vi "SnapShoot.vi"(8 "error in (no error)":errorcluster, 11 "ICameraTestingProxy in":refnum<class "ICameraTestingProxy.lvclass">) -> (0 "error out":errorcluster, 2 "SnapData":T1, 3 "ICameraTestingProxy out":refnum<class "ICameraTestingProxy.lvclass">)   [LabVIEW 2020, in "ICameraTestingProxy.lvlib" / "ICameraTestingProxy.lvclass"]
uses:
  ICameraTestingProxy.lvclass
  TypeDef/SnapData.ctl
  TypeDef/ICameraTestingProxy_typedef.lvlib
  TypeDef/Resolution.ctl
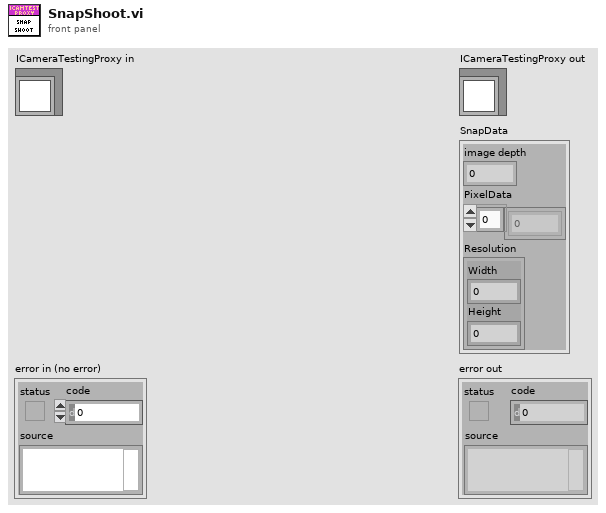
[diagram p1: front panel]
types:
  T1 = typedef "ICameraTestingProxy_typedef.lvlib/SnapData.ctl" = cluster{"image depth":i32, "PixelData":u8[], "Resolution":T2}
  T2 = typedef "ICameraTestingProxy_typedef.lvlib/Resolution.ctl" = cluster{"Width":i16, "Height":i16}
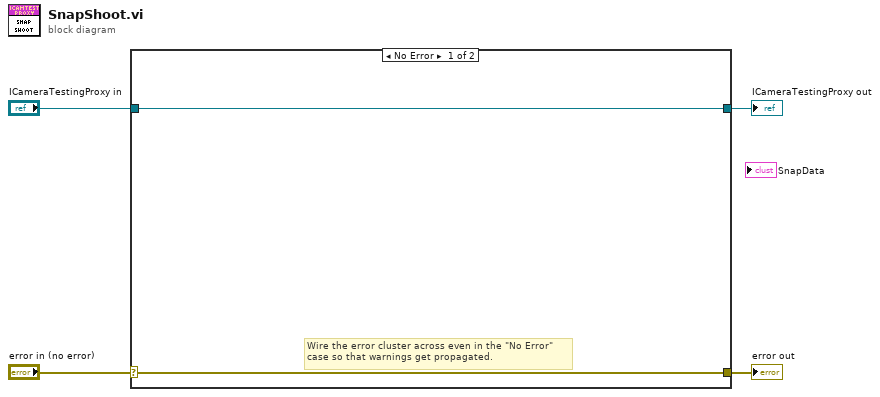
[diagram p0: block diagram]
diagram:
  n1 = case shown="No Error" "error in (no error)" {
    selector: "error in (no error)" -> [w5 w8]
    tunnel: [w5 w8] -> w3
    tunnel: [w6 w7] -> w1
    tunnel: "ICameraTestingProxy in" -> [w6 w7]
    frame No Error {
      # "Wire the error cluster across even in the \"No Error\"\ncase so that warnings get propagated."
    }
    frame Error {
    }
  }
  "error out" <- w3
  "ICameraTestingProxy out" <- w1
